vi "acquireValue.vi"(8 "error in (no error)":errorcluster, 10 "nextSample?":bool, 11 "loopTime in":refnum<class "loopTime.lvclass">) -> (0 "error out":errorcluster, 1 "function return":i32, 2 "variantData":variant, 3 "loopTime out":refnum<class "loopTime.lvclass">)   [LabVIEW 2016, in "SALLV_EXA_Messaging.lvlib" / "loopTime.lvclass"]
uses:
  loopTime.lvclass
  loopTime.lvclass/loopTime.ctl
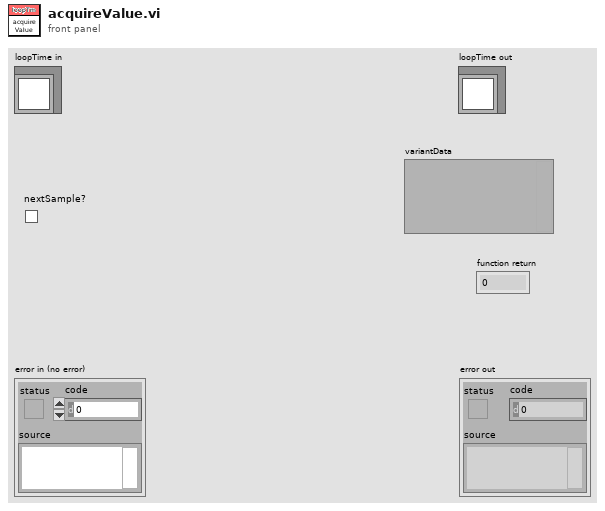
[diagram p1: front panel]
types:
  T1 = typedef "SALLV_EXA.lvlib/timestamp.ctl" = cluster{"timestamp":dbl}
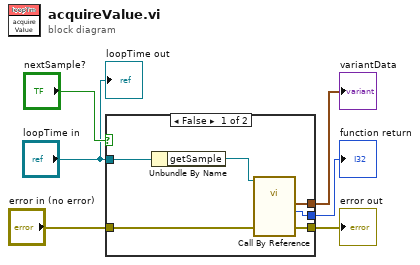
[diagram p0: block diagram]
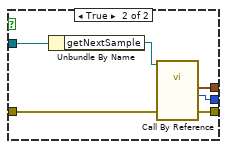
[diagram p2: hidden frame]
diagram:
  n1 = case shown="False" "nextSample?" {
    tunnel: "error in (no error)" -> [w10 w16]
    tunnel: [w9 w15] -> w2
    tunnel: [w7 w13] -> w3
    tunnel: [w8 w14] -> w4
    tunnel: "loopTime in" -> [w11 w18]
    frame False {
      n2 = Unbundle By Name(w11) -> ("getSample"=w12:refnum<vi>)
      n3 = call-by-ref "?"(reference=w12, "error in (no error)"=w10) -> ("error out"=w9:errorcluster, "function return"=w8:i32, "timestamp_Ctl out"=w7:T1)  [unwired: 9 in, 2 out]
    }
    frame True {
      n4 = Unbundle By Name(w18) -> ("getNextSample"=w17:refnum<vi>)
      n5 = call-by-ref "?"(reference=w17, "error in (no error)"=w16) -> ("error out"=w15:errorcluster, "function return"=w14:i32, "timestamp_Ctl out"=w13:T1)  [unwired: 9 in, 2 out]
    }
  }
  "error out" <- w2
  "variantData" <- w3
  "function return" <- w4
  "loopTime out" <- "loopTime in"
